vi "TESTE.vi"() -> ()   [LabVIEW 2018]
panel:
  out "Array":string[](array[string])
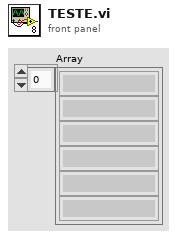
[diagram p1: front panel]
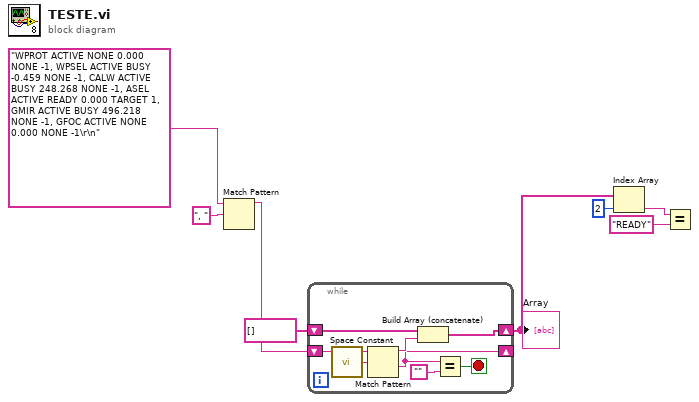
[diagram p0: block diagram]
diagram:
  n1 = Match Pattern(string="WPROT ACTIVE NONE 0.000 NONE -1, WPSEL ACTIVE BUSY -0.459 NONE -1, CALW ACTIVE BUSY 248.268 NONE -1, ASEL ACTIVE READY 0.000 TARGET 1, GMIR ACTIVE BUSY 496.218 NONE -1, GFOC ACTIVE NONE 0.000 NONE -1\r\n" ("search string/char (-)"), regular expression=", " ("search string/char (-)")) -> (before substring=w5:string)  [unwired: 1 in, 3 out]
  n2 = while {
    shift-right: [w13] -> w4
    shift-left: string[] [] -> [w14]
    shift-right: [w10] -> _
    shift-left: w5 -> [w12]
    stop <- w15 stop-if-true
    n3 = call <vilib>:"Space Constant.vi"() -> ("String"=w9:string)
    n4 = Match Pattern(string=w12, regular expression=w9) -> (before substring=w11:string, after substring=w10:string)  [unwired: 1 in, 2 out]
    n5 = Build Array (concatenate)(w14, w11) -> (w13:string[])
    n6 = Equal?(x=w10, y="") -> (x = y?=w15:bool)
  }
  "Array" <- w4
  n7 = Index Array(array=w4, index=2) -> (element=w2:string)
  n8 = Equal?(x=w2, y="READY") -> ()  [unwired: 1 out]
